vi "Configure IQ Recorder Measurement Format.vi"(8 "error in (no error)":errorcluster, 9 "Format (Cartesian Coordinates)":i32(ring) items=["Cartesian Coordinates", "Polar Coordinates"], 10 "Instance (1)":i32=1, 11 "VISA resource name":refnum<visa-resource-name>) -> (0 "error out":errorcluster, 3 "VISA resource name out":refnum<visa-resource-name>)   [LabVIEW 2020, in "Rohde&Schwarz CMXP GPRF.lvlib"]
doc: "This VI selects the coordinates that are used to represent the I/Q Recorder results.\n\nAttribute:\nRSCMXPGPRF_ATTR_IQ_RECORDER_MEASUREMENT_FORMAT\n\nRemote-control command:\nCONFigure:GPRF:MEAS<i>:IQRecorder:FORMat"
uses:
  <instrlib>/Rohde&Schwarz CMXP GPRF/Rohde&Schwarz CMXP GPRF.lvlib
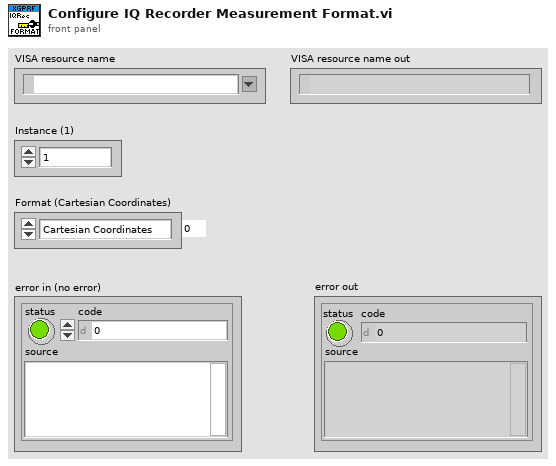
[diagram p1: front panel]
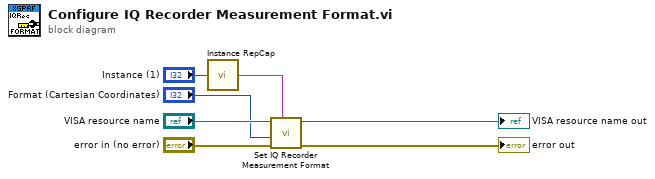
[diagram p0: block diagram]
diagram:
  n1 = call <instrlib>:"Instance RepCap.vi"("Instance in"="Instance (1)") -> ("Instance out"=w4:string)
  n2 = call "Set IQ Recorder Measurement Format"("Repeated Capabilities"=w4, "error in (no error)"="error in (no error)", "IQ Recorder Measurement Format (0 - Cartesian Coordinates)"="Format (Cartesian Coordinates)", "instrument handle"="VISA resource name") -> ("error out"=→"error out":errorcluster, "instrument handle out"=→"VISA resource name out":refnum<visa-resource-name>)  [unwired: 6 in]
